vi "Run.vi"(7 "Team Index":i32, 8 "Column":i32, 9 "Row":i32, 10 "View":i32[](array[numeric]) caption="View (Team Index, -1: empty)", 11 "Line Dancer in":refnum<class "Swirly Vortex of Terror.lvclass">) -> (0 "Replicated":refnum<class "Square.lvclass">, 1 "Direction":T1, 2 "Action":T2, 3 "Square Out":refnum<class "Square.lvclass">)   [LabVIEW 2015, in "Swirly Vortex of Terror.lvclass"]
uses:
  Swirly Vortex of Terror.lvclass
  Square/Square.lvclass
  Type Defs/Action Enum.ctl
  Type Defs/Direction Enum.ctl
  Common/Attack Options.ctl
  Swirly Vortex of Terror.lvclass/Swirly Vortex of Terror.ctl
  Type.ctl
  Common/Position.ctl
  SubVIs/Read-Only Globals.vi
  SubVIs/Globals (private).vi
  SubVIs/Read-Only Stats.vi
  Common/Find Enemy.vi
  Type Defs/SB Type Defs.lvlib
  Common/Common.lvlib
panel:
  # "NW\nN\nNE\nE\nSE\nS\nSW\nW"
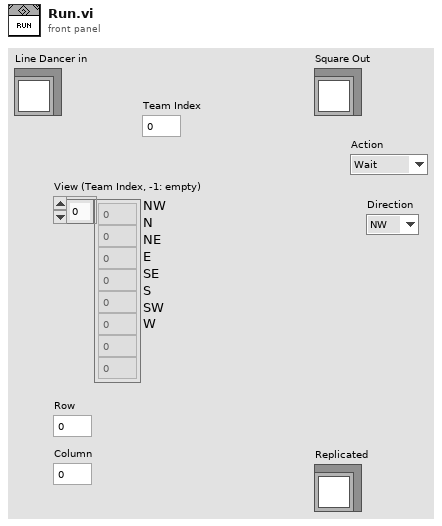
[diagram p1: front panel]
types:
  T1 = typedef "SB Type Defs.lvlib/Direction Enum.ctl" = enum16{"NW", "N", "NE", "E", "SE", "S", "SW", "W"}
  T2 = typedef "SB Type Defs.lvlib/Action Enum.ctl" = enum16{"Wait", "Move", "Attack", "Replicate"}
  T3 = typedef "Common.lvlib/Attack Options.ctl" = enum16{"Attack", "Run", "Distract"}
  T4 = typedef "Swirly Vortex of Terror.lvclass/Type.ctl" = enum16{"Diagonal Starter", "Row Starter", "Vortex Eye", "Disciple", "Path Keeper", "Explorer"}
  T5 = typedef "Common.lvlib/Position.ctl" = cluster{"Column":i32, "Row":i32}
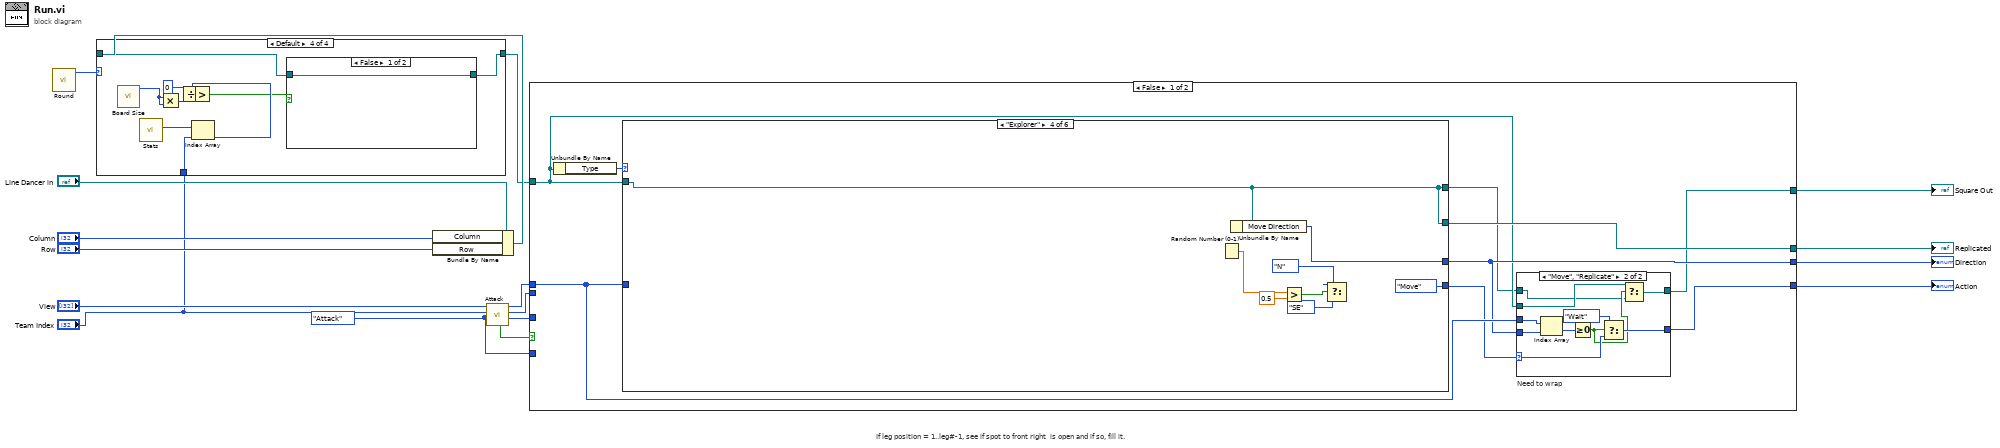
[diagram p0: block diagram]
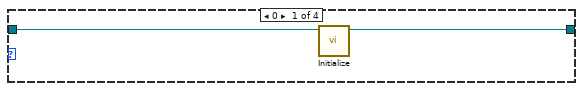
[diagram p2: hidden frame]
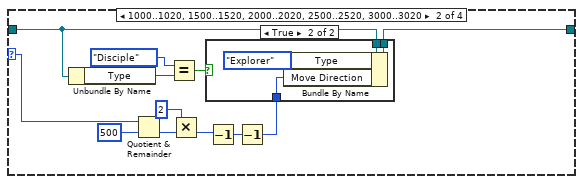
[diagram p3: hidden frame]
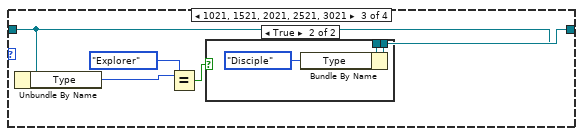
[diagram p5: hidden frame]
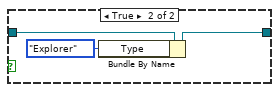
[diagram p7: hidden frame]
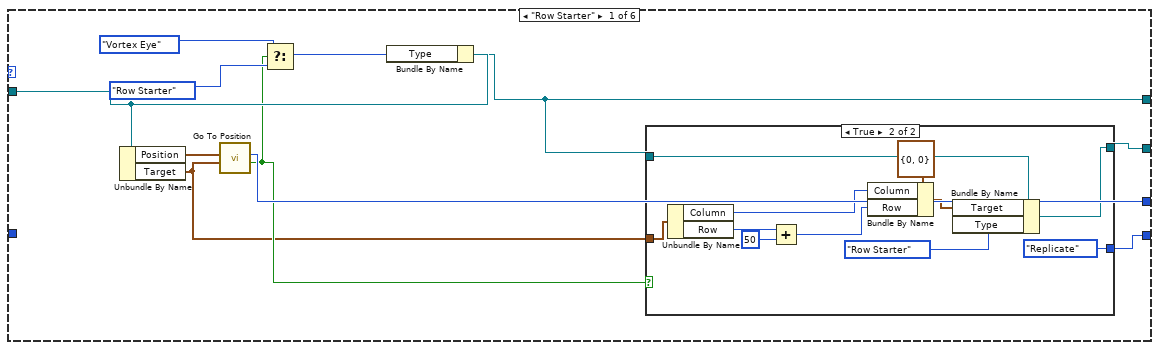
[diagram p9: hidden frame]
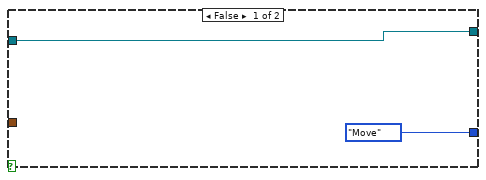
[diagram p10: hidden frame]
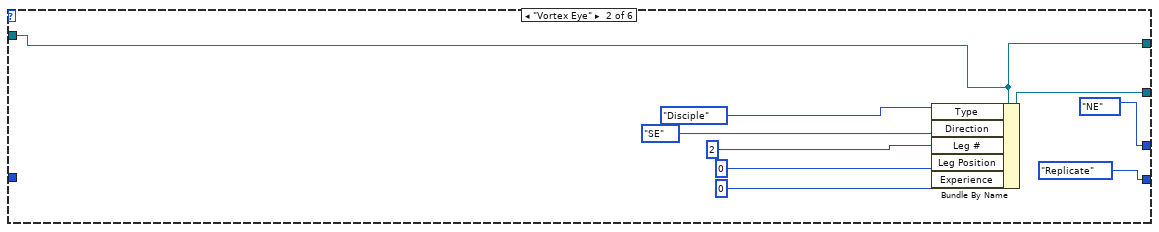
[diagram p11: hidden frame]
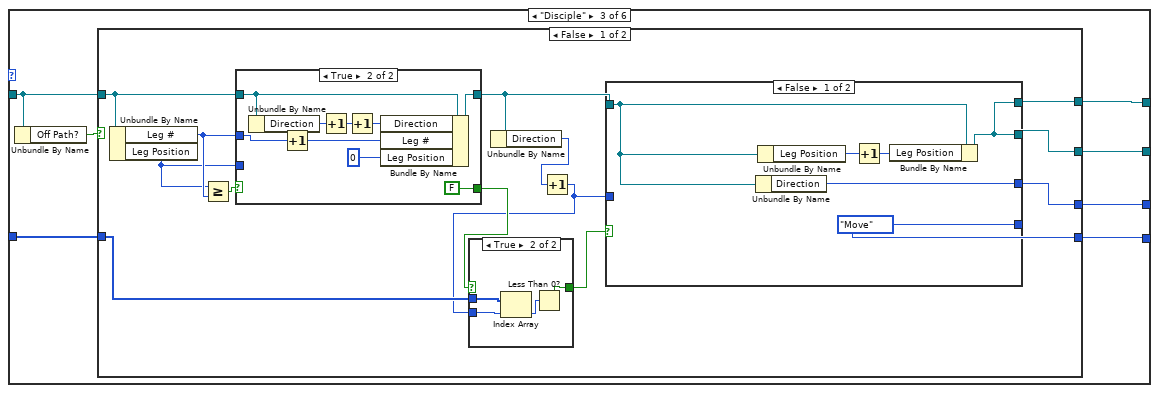
[diagram p12: hidden frame]
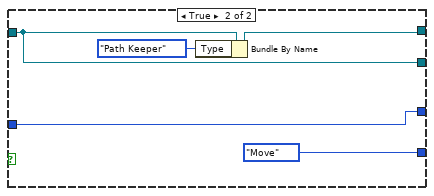
[diagram p14: hidden frame]
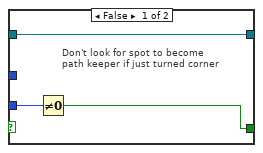
[diagram p15: hidden frame]
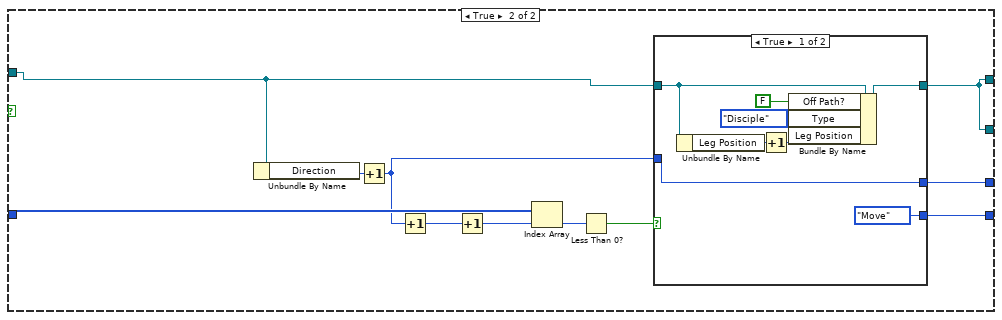
[diagram p16: hidden frame]
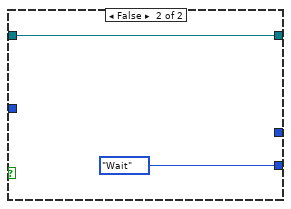
[diagram p17: hidden frame]
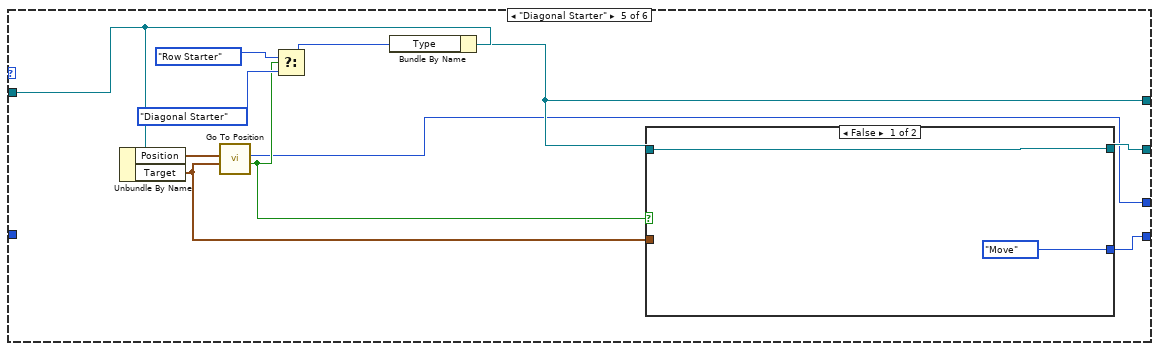
[diagram p18: hidden frame]
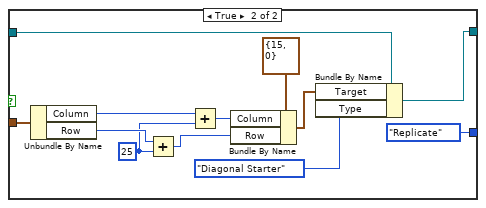
[diagram p19: hidden frame]
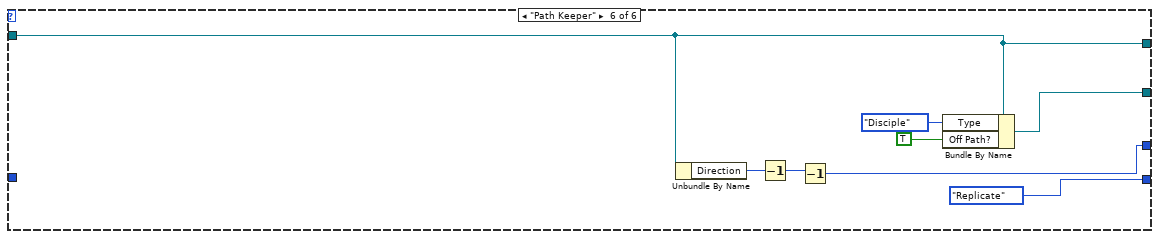
[diagram p20: hidden frame]
diagram:
  w2 = Attack_Options."Attack" ("Attack?")
  # "If leg position = 1..leg#-1, see if spot to front right  is open and if so, fill it."
  n1 = call "Round.vi"() -> ("Round"=w6:i32)  [unwired: 11 in]
  n2 = Bundle By Name(cluster="Line Dancer in", "Column"="Column", "Row"="Row") -> (w4:refnum<class "Swirly Vortex of Terror.lvclass">)
  n3 = case shown="Default" w6 {
    selector: w6 -> [_ w26 _ _]
    tunnel: w4 -> [w19 w30 w40 w48]
    tunnel: [w18 w31 w41 w47] -> w3
    tunnel: "Team Index" -> [_ _ _ w53]
    frame 0 {
      n4 = call "Initialize.vi"("Swirly Vortex of Terror In"=w19) -> ("Swirly Vortex of Terror Out"=w18:refnum<class "Swirly Vortex of Terror.lvclass">)  [unwired: 10 in]
    }
    frame 1000..1020, 1500..1520, 2000..2020, 2500..2520, 3000..3020 {
      n5 = Unbundle By Name(w30) -> ("Type"=w29:T4)
      n6 = Quotient & Remainder(x=w26, y=500) -> (floor(x/y)=w24:i32)  [unwired: 1 out]
      n7 = Equal?(x=Type."Disciple" ("y"), y=w29) -> (x = y?=w27:bool)
      n8 = Multiply(x=2, y=w24) -> (x*y=w23:i32)
      n9 = Decrement(x=w23) -> (x-1=w21:i32)
      n10 = Decrement(x=w21) -> (x-1=w20:i32)
      n11 = case shown="True" w27 {
        tunnel: [w32 w36] -> w31
        tunnel: w30 -> [w32 w34]
        tunnel: w20 -> [_ w33]
        frame False {
        }
        frame True {
          n12 = Bundle By Name(cluster=w34, "Type"=Type."Explorer" ("Player. Type"), "Move Direction"=w33) -> (w36:refnum<class "Swirly Vortex of Terror.lvclass">)
        }
      }
    }
    frame 1021, 1521, 2021, 2521, 3021 {
      n13 = Unbundle By Name(w40) -> ("Type"=w39:T4)
      n14 = Equal?(x=w39, y=Type."Explorer") -> (x = y?=w37:bool)
      n15 = case shown="True" w37 {
        tunnel: [w42 w45] -> w41
        tunnel: w40 -> [w42 w43]
        frame False {
        }
        frame True {
          n16 = Bundle By Name(cluster=w43, "Type"=Type."Disciple" ("Player. Type")) -> (w45:refnum<class "Swirly Vortex of Terror.lvclass">)
        }
      }
    }
    frame Default {
      n17 = call "Board Size.vi"() -> ("Board Size"=w55:i32)  [unwired: 11 in]
      n18 = call "Stats.vi"() -> ("Generated"=w46:i32[])  [unwired: 7 in, 4 out]
      n19 = Multiply(x=w55, y=w55) -> (x*y=w54:i32)
      n20 = Divide(x=w54, y=0 ("x")) -> (x/y=w51:dbl)
      n21 = Index Array(array=w46, index=w53) -> (element=w52:i32)
      n22 = Greater?(x=w52, y=w51) -> (0:w49:bool)
      n23 = case shown="False" w49 {
        tunnel: w48 -> [w56 w59]
        tunnel: [w56 w58] -> w47
        frame False {
        }
        frame True {
          n24 = Bundle By Name(cluster=w59, "Type"=Type."Explorer" ("Player. Type")) -> (w58:refnum<class "Swirly Vortex of Terror.lvclass">)
        }
      }
    }
  }
  n25 = call "Attack.vi"("Attack?"=w2, "Team Index"="Team Index", "View"="View") -> ("Direction"=w10:i32, "Action"=w11:T2, "View"=w13:i32[], "Enemy Found?"=w12:bool)  [unwired: 3 in, 2 out]
  n26 = case shown="False" w12 {
    tunnel: [w63 w228] -> w17
    tunnel: [w65 w227] -> w16
    tunnel: w3 -> [w62 w231]
    tunnel: [w60 w231] -> w15
    tunnel: [w68 w231] -> w14
    tunnel: w13 -> [w66 w230]
    tunnel: w11 -> [_ w229]
    tunnel: w10 -> [_ w226]
    tunnel: w2 -> [_ w225]
    frame False {
      # "Need to wrap"
      n27 = Unbundle By Name(w62) -> ("Type"=w67:T4)
      n28 = case shown="\"Explorer\"" w67 {
        tunnel: [w83 Action_Enum."Replicate" ("f") w119 Action_Enum."Move" ("f") w195 Action_Enum."Replicate" ("f")] -> w64
        tunnel: [w91 Direction_Enum."NE" ("Direction") w118 w184 w193 w218] -> w65
        tunnel: w66 -> [_ _ w120 _ _ _]
        tunnel: [w86 w110 w116 w185 w198 w222] -> w68
        tunnel: [w85 w111 w117 w185 w197 w221] -> w61
        tunnel: w62 -> [w88 w111 w115 w185 w200 w221]
        frame "Row Starter" {
          n29 = Unbundle By Name(w88) -> ("Position"=w87:T5, "Target"=w82:T5)
          n30 = call "Go To Position.vi"("Target Position"=w82, "My Position"=w87) -> ("Arrived?"=w84:bool, "Direction"=w91:T1)  [unwired: 7 in, 1 out]
          n31 = Select(t=Type."Vortex Eye" ("Player. Type"), s=w84, f=Type."Row Starter" ("Player. Type")) -> (s? t:f=w89:T4)
          n32 = Bundle By Name(cluster=w88, "Type"=w89) -> (w85:refnum<class "Swirly Vortex of Terror.lvclass">)
          n33 = case shown="True" w84 {
            tunnel: [w93 w96] -> w86
            tunnel: w85 -> [w93 w97]
            tunnel: [Action_Enum."Move" ("f") Action_Enum."Replicate" ("f")] -> w83
            tunnel: w82 -> [_ w98]
            frame False {
            }
            frame True {
              n34 = Unbundle By Name(w98) -> ("Column"=w95:i32, "Row"=w100:i32)
              n35 = Add(x=w100, y=50) -> (x+y=w103:i32)
              n36 = Bundle By Name(cluster=T5 {"Column"=0, "Row"=0} ("Target"), "Column"=w95, "Row"=w103) -> (w102:T5)
              n37 = Bundle By Name(cluster=w97, "Target"=w102, "Type"=Type."Row Starter" ("Player. Type")) -> (w96:refnum<class "Swirly Vortex of Terror.lvclass">)
            }
          }
        }
        frame "Vortex Eye" {
          n38 = Bundle By Name(cluster=w111, "Type"=Type."Disciple" ("Player. Type"), "Direction"=Direction_Enum."SE" ("Player.Direction"), "Leg #"=2 ("Player.Leg #"), "Leg Position"=0 ("Player.Leg Position"), "Experience"=0 ("Player.Experience")) -> (w110:refnum<class "Swirly Vortex of Terror.lvclass">)
        }
        frame "Disciple" {
          n39 = Unbundle By Name(w115) -> ("Off Path?"=w114:bool)
          n40 = case shown="False" w114 {
            tunnel: w120 -> [w125 w166]
            tunnel: [w134 w173] -> w119
            tunnel: w115 -> [w133 w168]
            tunnel: [w130 w169] -> w118
            tunnel: [w129 w167] -> w117
            tunnel: [w128 w167] -> w116
            frame False {
              n41 = Unbundle By Name(w133) -> ("Leg #"=w131:i32, "Leg Position"=w124:i32)
              n42 = Greater Or Equal?(x=w124, y=w131) -> (x >= y?=w132:bool)
              n43 = case shown="True" w132 {
                tunnel: [w153 w162] -> w123
                tunnel: w133 -> [w153 w161]
                tunnel: w131 -> [_ w159]
                tunnel: [w151 FALSE] -> w127
                tunnel: w124 -> [w152 _]
                frame False {
                  # "Don't look for spot to become\npath keeper if just turned corner"
                  n44 = Not Equal To 0?(x=w152) -> (x != 0?=w151:bool)
                }
                frame True {
                  n45 = Unbundle By Name(w161) -> ("Direction"=w160:T1)
                  n46 = Increment(x=w159) -> (x+1=w158:i32)
                  n47 = Increment(x=w160) -> (x+1=w156:T1)
                  n48 = Increment(x=w156) -> (x+1=w155:T1)
                  n49 = Bundle By Name(cluster=w161, "Direction"=w155, "Leg #"=w158, "Leg Position"=0 ("Player.Leg Position")) -> (w162:refnum<class "Swirly Vortex of Terror.lvclass">)
                }
              }
              n50 = Unbundle By Name(w123) -> ("Direction"=w122:T1)
              n51 = Increment(x=w122) -> (x+1=w121:T1)
              n52 = case shown="True" w127 {
                selector: w127 -> [w135 _]
                tunnel: [w135 w137] -> w126
                tunnel: w125 -> [_ w139]
                tunnel: w121 -> [_ w136]
                frame False {
                }
                frame True {
                  n53 = Index Array(array=w139, index=w136) -> (element=w138:i32)
                  n54 = Less Than 0?(x=w138) -> (x < 0?=w137:bool)
                }
              }
              n55 = case shown="False" w126 {
                tunnel: [Action_Enum."Move" ("f") Action_Enum."Move" ("f")] -> w134
                tunnel: [w142 w149] -> w128
                tunnel: w123 -> [w141 w149]
                tunnel: [w142 w148] -> w129
                tunnel: [w140 w146] -> w130
                tunnel: w121 -> [_ w146]
                frame False {
                  n56 = Unbundle By Name(w141) -> ("Direction"=w140:T1)
                  n57 = Unbundle By Name(w141) -> ("Leg Position"=w144:i32)
                  n58 = Increment(x=w144) -> (x+1=w143:i32)
                  n59 = Bundle By Name(cluster=w141, "Leg Position"=w143) -> (w142:refnum<class "Swirly Vortex of Terror.lvclass">)
                }
                frame True {
                  n60 = Bundle By Name(cluster=w149, "Type"=Type."Path Keeper" ("Player. Type")) -> (w148:refnum<class "Swirly Vortex of Terror.lvclass">)
                }
              }
            }
            frame True {
              n61 = Unbundle By Name(w168) -> ("Direction"=w171:T1)
              n62 = Increment(x=w171) -> (x+1=w163:T1)
              n63 = Increment(x=w163) -> (x+1=w172:T1)
              n64 = Increment(x=w172) -> (x+1=w164:T1)
              n65 = Index Array(array=w166, index=w164) -> (element=w170:i32)
              n66 = Less Than 0?(x=w170) -> (x < 0?=w165:bool)
              n67 = case shown="True" w165 {
                tunnel: [Action_Enum."Move" ("f") Action_Enum."Wait" ("f")] -> w173
                tunnel: [w180 _] -> w169
                tunnel: w163 -> [w180 _]
                tunnel: w168 -> [w176 w182]
                tunnel: [w179 w182] -> w167
                frame True {
                  n68 = Unbundle By Name(w176) -> ("Leg Position"=w175:i32)
                  n69 = Increment(x=w175) -> (x+1=w174:i32)
                  n70 = Bundle By Name(cluster=w176, "Off Path?"=FALSE ("Player.Off Path?"), "Type"=Type."Disciple" ("Player. Type"), "Leg Position"=w174) -> (w179:refnum<class "Swirly Vortex of Terror.lvclass">)
                }
                frame False {
                }
              }
            }
          }
        }
        frame "Explorer" {
          n71 = Random Number (0-1)() -> (number: 0 to 1=w190:dbl)
          n72 = Unbundle By Name(w185) -> ("Move Direction"=w184:T1)
          n73 = Greater?(x=w190, y=0.5) -> (0:w188:bool)
          n74 = Select(t=Direction_Enum."N", s=w188, f=Direction_Enum."SE") -> ()  [unwired: 1 out]
        }
        frame "Diagonal Starter" {
          n75 = Unbundle By Name(w200) -> ("Position"=w199:T5, "Target"=w194:T5)
          n76 = call "Go To Position.vi"("Target Position"=w194, "My Position"=w199) -> ("Arrived?"=w196:bool, "Direction"=w193:T1)  [unwired: 7 in, 1 out]
          n77 = Select(t=Type."Row Starter" ("Player. Type"), s=w196, f=Type."Diagonal Starter" ("Player. Type")) -> (s? t:f=w201:T4)
          n78 = Bundle By Name(cluster=w200, "Type"=w201) -> (w197:refnum<class "Swirly Vortex of Terror.lvclass">)
          n79 = case shown="False" w196 {
            tunnel: [w204 w206] -> w198
            tunnel: w197 -> [w204 w207]
            tunnel: [Action_Enum."Move" ("f") Action_Enum."Replicate" ("f")] -> w195
            tunnel: w194 -> [_ w208]
            frame False {
            }
            frame True {
              w205 = 25 ("y")
              n80 = Unbundle By Name(w208) -> ("Column"=w211:i32, "Row"=w214:i32)
              n81 = Add(x=w214, y=w205) -> (x+y=w215:i32)
              n82 = Add(x=w211, y=w205) -> (x+y=w213:i32)
              n83 = Bundle By Name(cluster=T5 {"Column"=15, "Row"=0} ("Target"), "Column"=w213, "Row"=w215) -> (w212:T5)
              n84 = Bundle By Name(cluster=w207, "Target"=w212, "Type"=Type."Diagonal Starter" ("Player. Type")) -> (w206:refnum<class "Swirly Vortex of Terror.lvclass">)
            }
          }
        }
        frame "Path Keeper" {
          n85 = Unbundle By Name(w221) -> ("Direction"=w219:T1)
          n86 = Decrement(x=w219) -> (x-1=w220:T1)
          n87 = Decrement(x=w220) -> (x-1=w218:T1)
          n88 = Bundle By Name(cluster=w221, "Type"=Type."Disciple" ("Player. Type"), "Off Path?"=TRUE ("Player.Off Path?")) -> (w222:refnum<class "Swirly Vortex of Terror.lvclass">)
        }
      }
      n89 = case shown="\"Move\", \"Replicate\"" w64 {
        selector: w64 -> [w70 w77]
        tunnel: w66 -> [_ w80]
        tunnel: w65 -> [_ w79]
        tunnel: [w70 w76] -> w63
        tunnel: w62 -> [_ w73]
        tunnel: w61 -> [w69 w72]
        tunnel: [w69 w71] -> w60
        frame Default {
        }
        frame "Move", "Replicate" {
          n90 = Index Array(array=w80, index=w79) -> (element=w78:i32)
          n91 = Greater Or Equal To 0?(x=w78) -> (x >= 0?=w74:bool)
          n92 = Select(t=Action_Enum."Wait", s=w74, f=w77) -> (s? t:f=w76:T2)
          n93 = Select(t=w73, s=w74, f=w72) -> (s? t:f=w71:refnum<class "Swirly Vortex of Terror.lvclass">)
        }
      }
    }
    frame True {
      n94 = case shown="\"Run\"" w225 {
        tunnel: w230 -> [_ w240]
        tunnel: w229 -> [w233 w238]
        tunnel: [w233 w236] -> w228
        tunnel: [w232 w235] -> w227
        tunnel: w226 -> [w232 w234]
        frame "Attack", Default {
        }
        frame "Run" {
          n95 = Index Array(array=w240, index=w234) -> (element=w239:i32)
          n96 = Less Than 0?(x=w239) -> (x < 0?=w237:bool)
          n97 = case shown="False" w237 {
            tunnel: w238 -> [_ w245]
            tunnel: [Action_Enum."Attack" ("Action") w245] -> w236
            tunnel: [w241 w244] -> w235
            tunnel: w234 -> [w242 w244]
            frame False {
              n98 = call "Reverse Direction.vi"("Direction in"=w242) -> ("Reverse Direction"=w241:i32)  [unwired: 10 in]
            }
            frame True {
            }
          }
        }
      }
    }
  }
  "Square Out" <- w15
  "Action" <- w17
  "Direction" <- w16
  "Replicated" <- w14
